vi "Logger_Path_Generated.vi"(8 "error in (no error)":errorcluster caption="错误输入（无错误）", 10 "LoggerKind":enum16{"软件上传日志", "软件其他日志", "软件错误日志", "软件监控日志"}(ring), 11 "Logger 输入":refnum<class "Logger.lvclass">) -> (0 "error out":errorcluster caption="错误输出", 2 "appended path":path, 3 "Logger 输出":refnum<class "Logger.lvclass">)   [LabVIEW 2019, in "Logger.lvclass"]
uses:
  <userlib>/Logger/Logger.lvclass
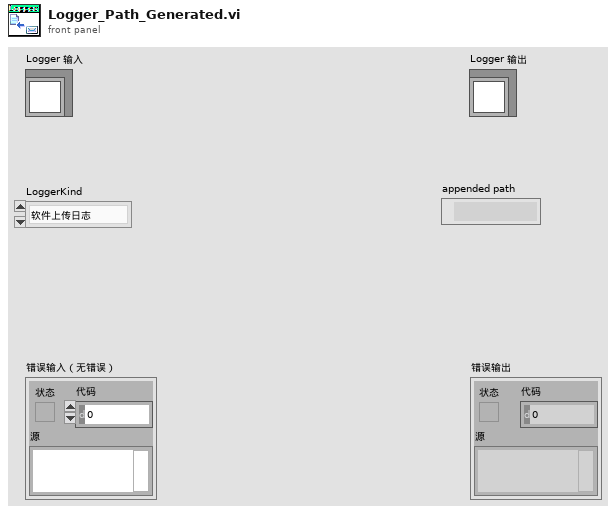
[diagram p1: front panel]
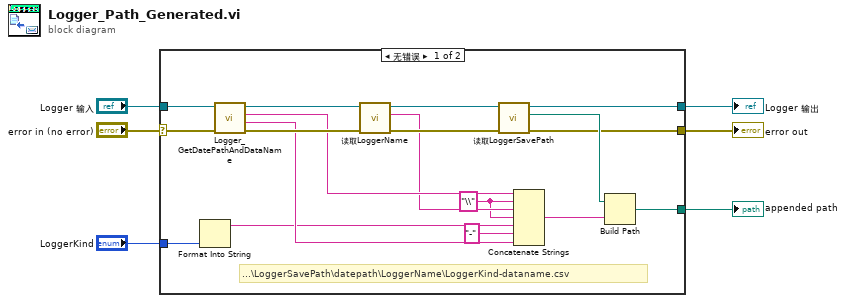
[diagram p0: block diagram]
diagram:
  n1 = case shown="无错误" "error in (no error)" {
    selector: "error in (no error)" -> [w18 w26]
    tunnel: [w20 w26] -> w5
    tunnel: [w22 w25] -> w3
    tunnel: "Logger 输入" -> [w19 w25]
    tunnel: [w9 _] -> w2
    tunnel: "LoggerKind" -> [w8 _]
    frame No Error {
      w13 = "\\" ("字符串")
      # "...\\LoggerSavePath\\datepath\\LoggerName\\LoggerKind-dataname.csv"
      n2 = Format Into String(w8) -> (resulting string=w7:string)  [unwired: 3 in, 1 out]
      n3 = call <userlib>:"Logger_GetDatePathAndDataName.vi"("error in (no error)"=w18, "Logger 输入"=w19) -> ("error out"=w16:errorcluster, "dataname"=w11:string, "datepath"=w15:string, "Logger 输出"=w17:refnum<class "Logger.lvclass">)  [unwired: 6 in]
      n4 = call "读取LoggerName.vi"("error in (no error)"=w16, "Logger输入"=w17) -> ("error out"=w21:errorcluster, "LoggerName"=w14:string, "Logger输出"=w24:refnum<class "Logger.lvclass">)  [unwired: 7 in]
      n5 = call "读取LoggerSavePath.vi"("error in (no error)"=w21, "Logger输入"=w24) -> ("error out"=w20:errorcluster, "LoggerSavePath"=w23:path, "Logger输出"=w22:refnum<class "Logger.lvclass">)  [unwired: 7 in]
      n6 = Concatenate Strings(w15, w13, w14, w13, w7, "-" ("字符串"), w11) -> (w10:string)
      n7 = Build Path(base path=w23, name or relative path=w10) -> (appended path=w9:path)
    }
    frame Error {
    }
  }
  "error out" <- w5
  "Logger 输出" <- w3
  "appended path" <- w2
